vi "05_DS_Augmentation_By_Flip_Rotate_By_Img.vi"() -> ()   [LabVIEW 2020]
uses:
  <vilib>/vision/NI_Vision_Development_Module.lvlib
panel:
  out "Progress":i32=429
  out "Total":i32=430
  in  "Image Path":path=path "D:/DNN/_AD/_from_Customers/2025_04_11_NIConnect_PCB5/1_Dataset/11_Augx4_Hue/Train"
  in  "Flip/Rotate Selector":enum16{"R180", "R_90/180/270"}(ring)
  out "error out":errorcluster
  in  "Image Type":T1=4 items=["Grayscale (U8)", "Grayscale (I16)", "Grayscale (SGL)", "Complex (CSG)", "RGB (U32)", "HSL (U32)", "RGB (U64)", "Grayscale (U16)"]
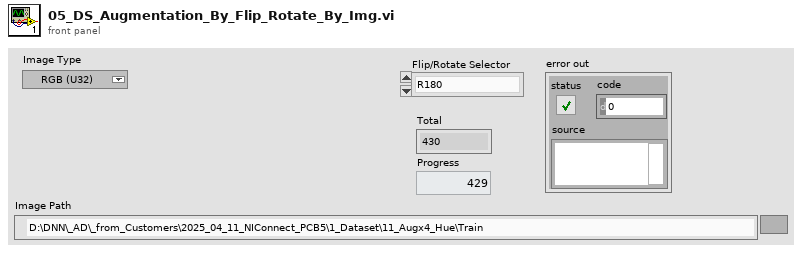
[diagram p1: front panel]
types:
  T1 = typedef "Image Type" = u32
  T2 = typedef "IMAQ Image.ctl" = refnum<image>
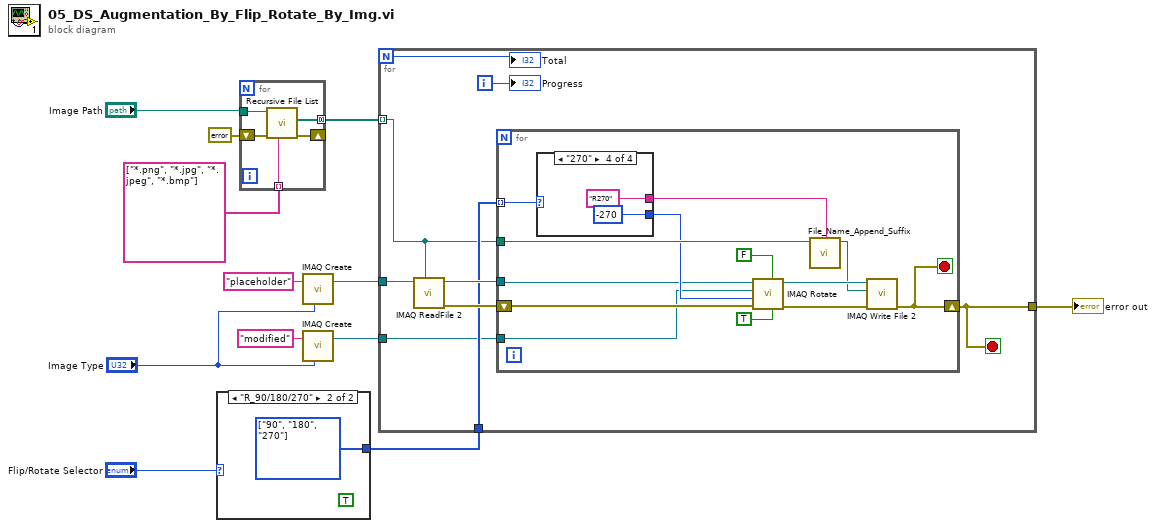
[diagram p0: block diagram]
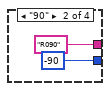
[diagram p3: hidden frame]
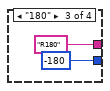
[diagram p4: hidden frame]
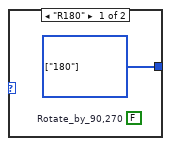
[diagram p5: hidden frame]
diagram:
  n1 = case shown="\"R_90/180/270\"" "Flip/Rotate Selector" {
    tunnel: [w13 w14] -> w7
    frame "R180" {
      (unwired) FALSE  # Rotate_by_90,270
      w13 = enum16{"0", "90", "180", "270"}[] [enum."180"] items=["0", "90", "180", "270"]
    }
    frame "R_90/180/270" {
      (unwired) TRUE ("Rotate_by_90,270")
      w14 = enum16{"0", "90", "180", "270"}[] [enum."90", enum."180", enum."270"] items=["0", "90", "180", "270"]
    }
  }
  n2 = for {
    tunnel: "Image Path" -> [w19]
    tunnel: string[] ["*.png", "*.jpg", "*.jpeg", "*.bmp"] ("pattern") -> [w18] mode=indexing
    tunnel: [w17] -> w2 mode=concatenating
    shift-right: [w15] -> _
    shift-left: errorcluster {"status"=FALSE, "code"=0, "source"=""} ("error out") -> [w16]
    n3 = call <vilib>:"Recursive File List.vi"("pattern"=w18, "error in (no error)"=w16, "Folder Path"=w19) -> ("error out"=w15:errorcluster, "All Files in Dir"=w17:path[])  [unwired: 4 in, 3 out]
  }
  n4 = call "IMAQ Create"("Image Name"="placeholder", "Image Type"="Image Type") -> ("New Image"=w11:T2)  [unwired: 3 in, 1 out]
  n5 = call "IMAQ Create"("Image Name"="modified", "Image Type"="Image Type") -> ("New Image"=w10:T2)  [unwired: 3 in, 1 out]
  n6 = for {
    N -> [w28]
    tunnel: w11 -> [w27]
    tunnel: w10 -> [w21]
    tunnel: w7 -> [w23]
    tunnel: [w25] -> w6
    tunnel: w2 -> [w22] mode=indexing
    i -> [w20]
    stop <- w25 stop-if-true
    n7 = call "IMAQ ReadFile 2"("File Path"=w22, "Image"=w27) -> ("error out"=w26:errorcluster, "Image Out"=w24:T2)  [unwired: 5 in, 3 out]
    n8 = for {
      tunnel: w23 -> [w39] mode=indexing
      tunnel: w24 -> [w32]
      tunnel: w22 -> [w38]
      shift-right: [w29] -> w25
      shift-left: w26 -> [w36]
      tunnel: w21 -> [w31]
      stop <- w29 stop-if-true
      n9 = case shown="\"270\"" w39 {
        tunnel: [_ "R090" "R180" "R270"] -> w34
        tunnel: [_ -90 -180 -270] -> w33
        frame "0", Default {
        }
        frame "90" {
        }
        frame "180" {
        }
        frame "270" {
        }
      }
      n10 = call "IMAQ Rotate"("Use Bilinear Interpolation"=TRUE, "Maintain Size"=FALSE, "error in (no error)"=w36, "Angle (degrees)"=w33, "Image Dst"=w31, "Image Src"=w32) -> ("error out"=w35:errorcluster, "Image Dst Out"=w40:T2)  [unwired: 4 in]
      n11 = call "File_Name_Append_Suffix.vi"("Suffix"=w34, "Path"=w38) -> ("appended path"=w37:path)  [unwired: 9 in]
      n12 = call-poly "IMAQ Write File 2"("error in (no error)"=w35, "File Path"=w37, "Image"=w40) -> ("error out"=w29:errorcluster)  [unwired: 7 in, 1 out]
    }
    "Total" <- w28
    "Progress" <- w20
  }
  "error out" <- w6
